vi "Get Steering Frame.vi"(8 "error in (no error)":errorcluster, 11 "ROV in":refnum<class "ROV Host.lvclass">) -> (0 "error out":errorcluster, 3 "ROV out":refnum<class "ROV Host.lvclass">, 4 "Teleop command":T1)   [LabVIEW 2012, in "ROV Host.lvclass"]
uses:
  ROV Host.lvclass
  Support/Teleop command.ctl
  ROV Host.lvclass/ROV Host.ctl
  <vilib>/robotics/Steering/Steering Frame/NI_Robotics_Steering Frame.lvclass/NI_Robotics_Steering Frame.ctl
  <vilib>/robotics/Steering/Steering Frame/NI_Robotics_Steering Frame.lvclass
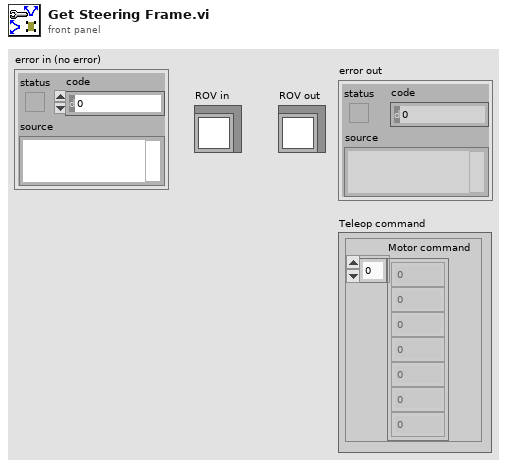
[diagram p1: front panel]
types:
  T1 = typedef "Teleop command.ctl" = cluster{"Motor command":dbl[]}
  T2 = typedef "NI_Robotics_Steering Class Types.lvlib/Mecanum Steering Frame.ctl" = refnum<class "NI_Robotics_Mecanum Steering Frame.lvclass">
  T3 = typedef "NI_Robotics_Steering Class Types.lvlib/Differential Steering Frame.ctl" = refnum<class "NI_Robotics_Differential Steering Frame.lvclass">
  T4 = typedef "NI_Robotics_Wheel.lvclass/Wheel State.ctl" = cluster{"wheel name":string, "forward angular velocity":dbl, "caster angular velocity":dbl, "caster wheel angle (rad)":dbl, "steering angle (rad)":dbl}
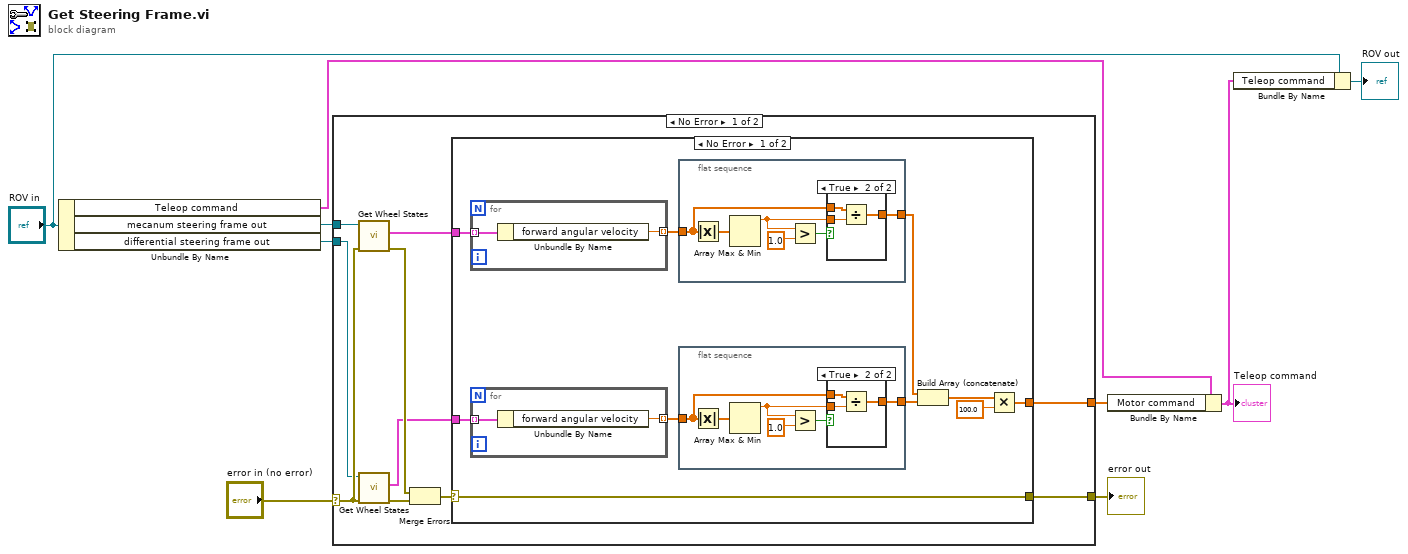
[diagram p0: block diagram]
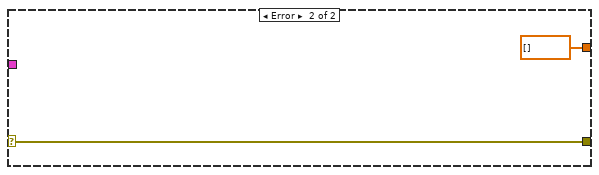
[diagram p4: hidden frame]
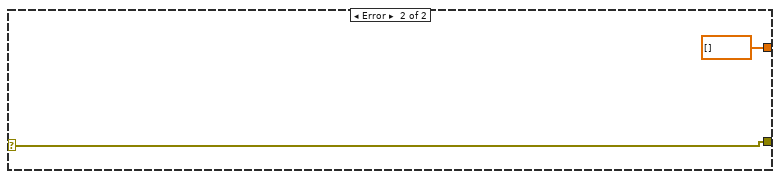
[diagram p5: hidden frame]
diagram:
  n1 = Unbundle By Name("ROV in") -> ("Teleop command"=w4:cluster{"Motor command":dbl[]}, "mecanum steering frame out"=w6:T2, "differential steering frame out"=w5:T3)
  n2 = case shown="No Error" "error in (no error)" {
    selector: "error in (no error)" -> [w17 w57]
    tunnel: [w13 w57] -> w7
    tunnel: w6 -> [w12 _]
    tunnel: w5 -> [w11 _]
    tunnel: [w10 dbl[] []] -> w3
    frame No Error {
      n3 = call <vilib>:"Get Wheel States.vi"("error in (no error)"=w17, "steering frame in"=w12) -> ("error out"=w18:errorcluster, "wheel states"=w15:T4[])  [unwired: 7 in, 1 out]
      n4 = call <vilib>:"Get Wheel States.vi"("error in (no error)"=w17, "steering frame in"=w11) -> ("error out"=w19:errorcluster, "wheel states"=w14:T4[])  [unwired: 7 in, 1 out]
      n5 = Merge Errors(w18, w19) -> (w16:errorcluster)
      n6 = case shown="No Error" w16 {
        selector: w16 -> [w29 w55]
        tunnel: w15 -> [w28 _]
        tunnel: w14 -> [w27 _]
        tunnel: [w29 w55] -> w13
        tunnel: [w21 dbl[] []] -> w10
        frame No Error {
          n7 = for {
            tunnel: w28 -> [w52] mode=indexing
            tunnel: [w53] -> w24 mode=indexing
            n8 = Unbundle By Name(w52) -> ("forward angular velocity"=w53:dbl)
          }
          n9 = for {
            tunnel: w27 -> [w50] mode=indexing
            tunnel: [w51] -> w26 mode=indexing
            n10 = Unbundle By Name(w50) -> ("forward angular velocity"=w51:dbl)
          }
          n11 = flat-sequence {
            tunnel: w24 -> [w33]
            tunnel: [w31] -> w23
            frame #0 {
              n12 = Absolute Value(x=w33) -> (abs(x)=w35:dbl[])
              n13 = Array Max & Min(array=w35) -> (max value=w32:dbl)  [unwired: 3 out]
              n14 = Greater?(x=w32, y=1.0) -> (0:w34:bool)
              n15 = case shown="True" w34 {
                tunnel: w33 -> [w36 w39]
                tunnel: w32 -> [_ w38]
                tunnel: [w36 w37] -> w31
                frame False {
                }
                frame True {
                  n16 = Divide(x=w39, y=w38) -> (x/y=w37:dbl[])
                }
              }
            }
          }
          n17 = flat-sequence {
            tunnel: w26 -> [w42]
            tunnel: [w40] -> w25
            frame #0 {
              n18 = Absolute Value(x=w42) -> (abs(x)=w45:dbl[])
              n19 = Array Max & Min(array=w45) -> (max value=w41:dbl)  [unwired: 3 out]
              n20 = Greater?(x=w41, y=1.0) -> (0:w43:bool)
              n21 = case shown="True" w43 {
                tunnel: w42 -> [w46 w49]
                tunnel: w41 -> [_ w48]
                tunnel: [w46 w47] -> w40
                frame False {
                }
                frame True {
                  n22 = Divide(x=w49, y=w48) -> (x/y=w47:dbl[])
                }
              }
            }
          }
          n23 = Build Array (concatenate)(w23, w25) -> (w22:dbl[])
          n24 = Multiply(x=w22, y=100.0) -> (x*y=w21:dbl[])
        }
        frame Error {
        }
      }
    }
    frame Error {
    }
  }
  "error out" <- w7
  n25 = Bundle By Name(cluster=w4, "Motor command"=w3) -> (w2:cluster{"Motor command":dbl[]})
  "Teleop command" <- w2
  n26 = Bundle By Name(cluster="ROV in", "Teleop command"=w2) -> (→"ROV out":refnum<class "ROV Host.lvclass">)
